vi "ROI grp-window queue interface.vi"() -> (0 "error out":errorcluster, 3 "ROI grouping window queue":refnum<queue>)   [LabVIEW 2013]
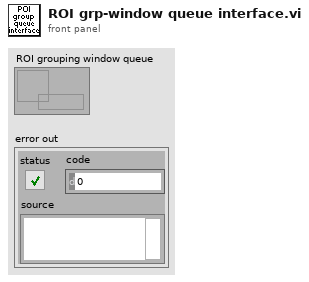
[diagram p1: front panel]
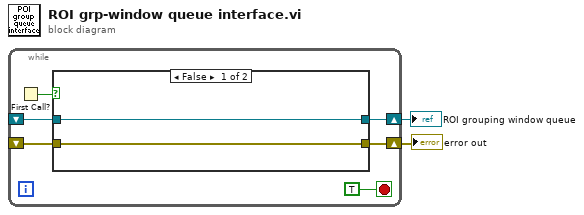
[diagram p0: block diagram]
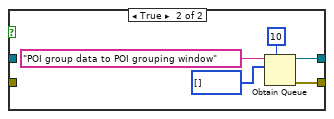
[diagram p2: hidden frame]
diagram:
  n1 = while {
    shift-right: [w6] -> w1
    shift-left: _ -> [w5]
    shift-right: [w4] -> w2
    shift-left: _ -> [w3]
    stop <- TRUE stop-if-true
    n2 = First Call?() -> (First Call?: T/F=w7:bool)
    n3 = case shown="False" w7 {
      tunnel: [w10 w12] -> w6
      tunnel: w5 -> [w10 _]
      tunnel: [w9 w11] -> w4
      tunnel: w3 -> [w9 _]
      frame False {
      }
      frame True {
        n4 = Obtain Queue(max queue size (-1, unlimited)=10, name (unnamed)="POI group data to POI grouping window", element data type=i32[] [] ("POI#")) -> (queue out=w12:refnum<queue>, error out=w11:errorcluster)  [unwired: 2 in, 1 out]
      }
    }
  }
  "ROI grouping window queue" <- w1
  "error out" <- w2
